vi "start led experiment.vi"(5 "logarithmic output?":bool, 6 "output2 enabled":bool, 7 "output1 enabled":bool, 8 "error in":errorcluster, 9 "file name 2 ref":refnum<vi>, 10 "file name 1 ref":refnum<vi>, 11 "Teensy Serial Port":refnum<visa-resource-name>) -> (0 "error out":errorcluster, 2 "commands and responses":string, 3 "teensy serial port out":refnum<visa-resource-name>)   [LabVIEW 2013]
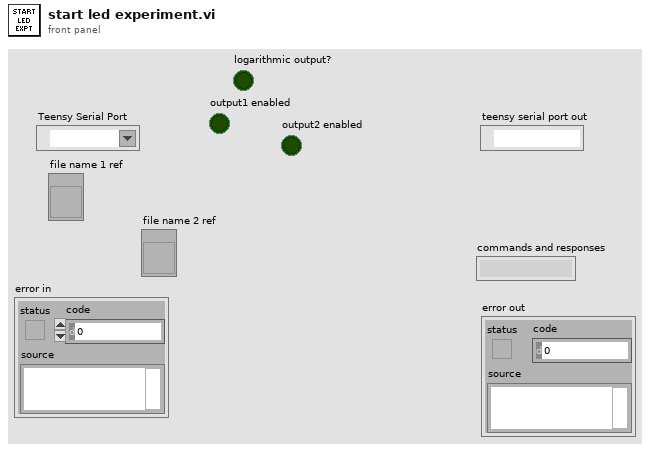
[diagram p1: front panel]
types:
  T1 = enum16{"R - open file for Reading", "W - open file for Writing", "S - send bytes", "F - fetch bytes", "B - begin experiment", "E - end experiment", "N - set number of bits per frame", "I - get info", "Q - Quiet (only error msgs)", "L - Loud (acknowledge all)", "T - set stimulus state", "Y - ready to start experiment", "H - useless Help message", "C - Close file", "O - enable/disable output", "G - set logarithmic output"}
  T2 = enum16{"R - open file for Reading", "W - open file for Writing", "S - send bytes", "F - fetch bytes", "B - begin experiment", "E - end experiment", "N - set number of bits per frame", "I - get info", "Q - Quiet (only error msgs)", "L - Loud (acknowledge all)", "T - set stimulus state", "Y - ready to start experiment", "H - useless Help message", "C - Close file"}
  T3 = enum16{"R - open file for Reading", "W - open file for Writing", "S - send bytes", "F - fetch bytes", "B - begin experiment", "E - end experiment", "N - set number of bits per frame", "I - get info", "Q - Quiet (only error msgs)", "L - Loud (acknowledge all)", "T - set stimulus state", "Y - ready to start experiment", "H - useless Help message"}
  T4 = enum16{"R - open file for Reading", "W - open file for Writing", "S - send bytes", "F - fetch bytes", "B - begin experiment", "E - end experiment", "N - set number of bits per frame", "I - get info", "Q - Quiet (only error msgs)", "L - Loud (acknowledge all)", "T - set stimulus state", "Y - ready to start experiment", "H - useless Help message", "C - Close file", "O - enable/disable output"}
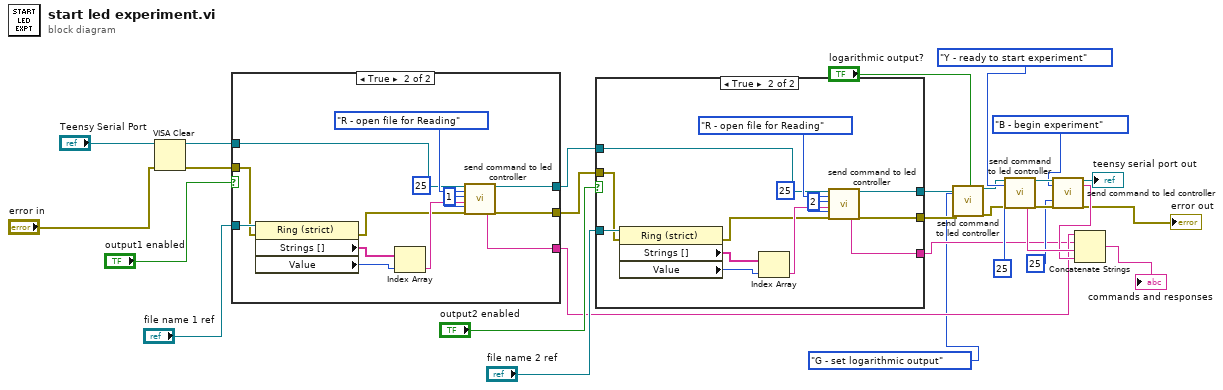
[diagram p0: block diagram]
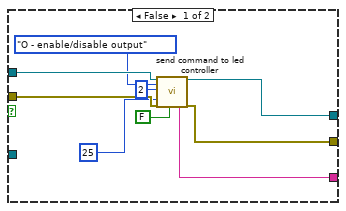
[diagram p2: hidden frame]
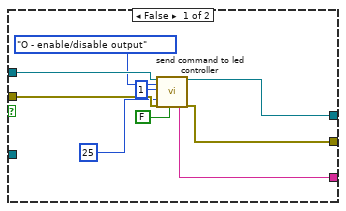
[diagram p3: hidden frame]
diagram:
  n1 = VISA Clear(VISA resource name="Teensy Serial Port", error in (no error)="error in") -> (VISA resource name out=w18:refnum<visa-resource-name>, error out=w16:errorcluster)
  n2 = case shown="True" "output1 enabled" {
    tunnel: [w38 w51] -> w11
    tunnel: [w37 w50] -> w12
    tunnel: [w30 w48] -> w8
    tunnel: "file name 1 ref" -> [_ w47]
    tunnel: w18 -> [w36 w42]
    tunnel: w16 -> [w35 w41]
    frame False {
      n3 = call "send command to led controller.vi"("Teensy Serial Port"=w36, "Command"=T4."O - enable/disable output", "lednumber"=u8 1, "milliseconds to wait between write and read"=u32 25, "error in"=w35, "output enabled"=FALSE) -> ("command and response with time"=w30:string, "teensy serial port out"=w37:refnum<visa-resource-name>, "error out"=w38:errorcluster)  [unwired: 8 in, 3 out]
    }
    frame True {
      n4 = property class="Ring (strict)"(reference=w47, error in=w41) -> (error out=w43:errorcluster, "Strings []"=w46:string[], "Value"=w45:u16)  [unwired: 1 out]
      n5 = Index Array(array=w46, index=w45) -> (element=w44:string)
      n6 = call "send command to led controller.vi"("Teensy Serial Port"=w42, "Command"=T2."R - open file for Reading", "lednumber"=u8 1, "milliseconds to wait between write and read"=u32 25, "error in"=w43, "file name"=w44) -> ("command and response with time"=w48:string, "teensy serial port out"=w50:refnum<visa-resource-name>, "error out"=w51:errorcluster)  [unwired: 8 in, 3 out]
    }
  }
  n7 = case shown="True" "output2 enabled" {
    tunnel: [w60 w73] -> w6
    tunnel: [w59 w72] -> w4
    tunnel: [w52 w70] -> w7
    tunnel: "file name 2 ref" -> [_ w69]
    tunnel: w12 -> [w58 w64]
    tunnel: w11 -> [w57 w63]
    frame False {
      n8 = call "send command to led controller.vi"("Teensy Serial Port"=w58, "Command"=T4."O - enable/disable output", "lednumber"=u8 2, "milliseconds to wait between write and read"=u32 25, "error in"=w57, "output enabled"=FALSE) -> ("command and response with time"=w52:string, "teensy serial port out"=w59:refnum<visa-resource-name>, "error out"=w60:errorcluster)  [unwired: 8 in, 3 out]
    }
    frame True {
      n9 = property class="Ring (strict)"(reference=w69, error in=w63) -> (error out=w65:errorcluster, "Strings []"=w68:string[], "Value"=w67:u16)  [unwired: 1 out]
      n10 = Index Array(array=w68, index=w67) -> (element=w66:string)
      n11 = call "send command to led controller.vi"("Teensy Serial Port"=w64, "Command"=T2."R - open file for Reading", "lednumber"=u8 2, "milliseconds to wait between write and read"=u32 25, "error in"=w65, "file name"=w66) -> ("command and response with time"=w70:string, "teensy serial port out"=w72:refnum<visa-resource-name>, "error out"=w73:errorcluster)  [unwired: 8 in, 3 out]
    }
  }
  n12 = call "send command to led controller.vi"("Teensy Serial Port"=w4, "Command"=T1."G - set logarithmic output", "error in"=w6, "logarithmic output?"="logarithmic output?") -> ("teensy serial port out"=w3:refnum<visa-resource-name>, "error out"=w5:errorcluster)  [unwired: 10 in, 4 out]
  n13 = call "send command to led controller.vi"("Teensy Serial Port"=w3, "Command"=T2."Y - ready to start experiment", "milliseconds to wait between write and read"=u32 25, "error in"=w5) -> ("command and response with time"=w26:string, "teensy serial port out"=w28:refnum<visa-resource-name>, "error out"=w29:errorcluster)  [unwired: 10 in, 3 out]
  n14 = call "send command to led controller.vi"("Teensy Serial Port"=w28, "Command"=T3."B - begin experiment", "milliseconds to wait between write and read"=u32 25, "error in"=w29) -> ("teensy serial port out"=→"teensy serial port out":refnum<visa-resource-name>, "response"=w25:string, "error out"=→"error out":errorcluster)  [unwired: 10 in, 3 out]
  n15 = Concatenate Strings(w8, w7, w26, w25) -> (→"commands and responses":string)
